vi "Coord window-Menu selection handler.vi"(11 "ItemTag":string) -> (0 "error out":errorcluster)   [LabVIEW 2013]
uses:
  Visualisation/Functional Imaging Viewer/SubVIs/Experiment header interface/Typedefs/Save-Load-Save as-Load last enum.ctl
  Globals/Coord window-Globals.vi
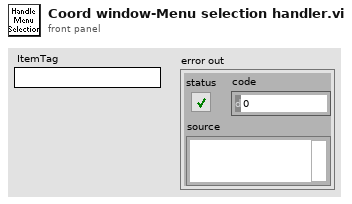
[diagram p1: front panel]
types:
  T1 = typedef "Save-Load-Save as-Load last enum.ctl" = enum16{"Save file", "Save file as", "Load file", "Load last file"}
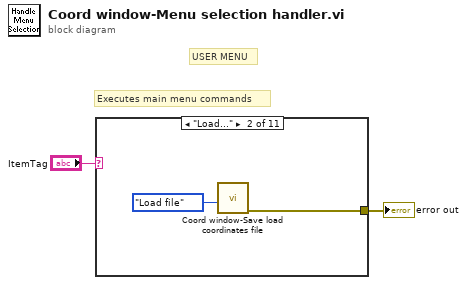
[diagram p0: block diagram]
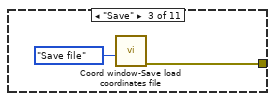
[diagram p3: hidden frame]
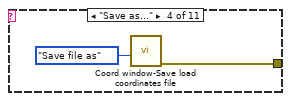
[diagram p4: hidden frame]
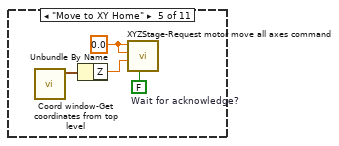
[diagram p5: hidden frame]
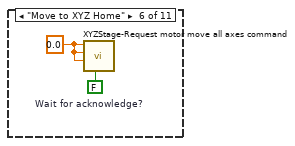
[diagram p6: hidden frame]
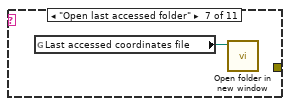
[diagram p7: hidden frame]
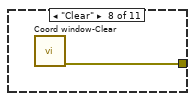
[diagram p8: hidden frame]
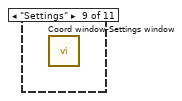
[diagram p9: hidden frame]
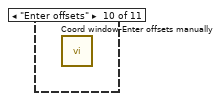
[diagram p10: hidden frame]
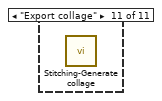
[diagram p11: hidden frame]
diagram:
  # "USER MENU"
  # "Executes main menu commands"
  n1 = case shown="\"Load...\"" "ItemTag" {
    tunnel: [_ w4 w6 w8 _ _ _ w16 _ _ _] -> w1
    frame Default {
    }
    frame "Load..." {
      n2 = call "Coord window-Save load coordinates file.vi"("Function"=Save-Load-Save_as-Load_last_enum."Load file") -> ("error out"=w4:errorcluster)  [unwired: 10 in]
    }
    frame "Save" {
      n3 = call "Coord window-Save load coordinates file.vi"("Function"=Save-Load-Save_as-Load_last_enum."Save file") -> ("error out"=w6:errorcluster)  [unwired: 10 in]
    }
    frame "Save as..." {
      n4 = call "Coord window-Save load coordinates file.vi"("Function"=Save-Load-Save_as-Load_last_enum."Save file as") -> ("error out"=w8:errorcluster)  [unwired: 10 in]
    }
    frame "Move to XY Home" {
      w12 = FALSE  # Wait for acknowledge?
      w11 = sgl 0.0 ("Motor X")
      n5 = call "Coord window-Get coordinates from top level.vi"() -> ("Coordinates"=w9:cluster{"X":sgl, "Y":sgl, "Z":sgl})  [unwired: 11 in]
      n6 = Unbundle By Name(w9) -> ("Z"=w10:sgl)
      n7 = call "XYZStage-Request motor move all axes command.vi"("Wait for acknowledge?"=w12, "Motor Z"=w10, "Motor Y"=w11, "Motor X"=w11) -> ()  [unwired: 6 in, 2 out]
    }
    frame "Move to XYZ Home" {
      w14 = FALSE  # Wait for acknowledge?
      w13 = sgl 0.0 ("Motor X")
      n8 = call "XYZStage-Request motor move all axes command.vi"("Wait for acknowledge?"=w14, "Motor Z"=w13, "Motor Y"=w13, "Motor X"=w13) -> ()  [unwired: 6 in, 2 out]
    }
    frame "Open last accessed folder" {
      n9 = global read "Coord window-Globals.vi" "Last accessed coordinates file"() -> (w15:path)
      n10 = call "Open folder in new window.vi"("Directory to open"=w15) -> ()  [unwired: 10 in, 1 out]
    }
    frame "Clear" {
      n11 = call "Coord window-Clear.vi"() -> ("error out"=w16:errorcluster)  [unwired: 11 in]
    }
    frame "Settings" {
      n12 = call "Coord window-Settings window.vi"() -> ()  [unwired: 11 in, 1 out]
    }
    frame "Enter offsets" {
      n13 = call "Coord window-Enter offsets manually.vi"() -> ()  [unwired: 11 in, 1 out]
    }
    frame "Export collage" {
      n14 = call "Stitching-Generate collage.vi"() -> ()  [unwired: 12 in]
    }
  }
  "error out" <- w1
